vi "Separar ejes serial.vi"(8 "error in":errorcluster, 11 "Read buffer":string) -> (0 "error out":errorcluster, 1 "Pos Z":i32, 2 "Pos Y":i32, 3 "Pos X":i32)   [LabVIEW 2021]
panel:
  out "Eje Z":string
  out "Eje Y":string
  out "Eje X":string
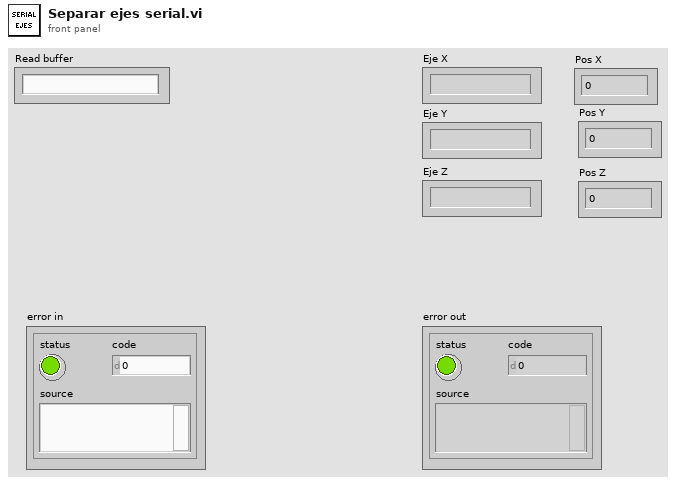
[diagram p1: front panel]
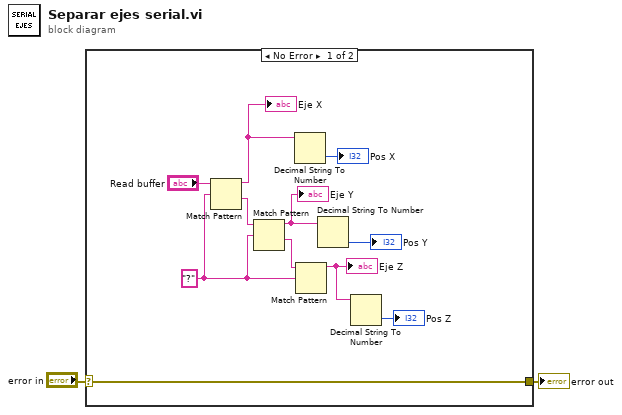
[diagram p0: block diagram]
diagram:
  n1 = case shown="No Error" "error in" {
    selector: "error in" -> [w13 w14]
    tunnel: [w13 w14] -> w1
    frame No Error {
      w9 = "?" ("regular expression")
      n2 = Match Pattern(string="Read buffer", regular expression=w9) -> (before substring=w8:string, after substring=w11:string)  [unwired: 1 in, 2 out]
      "Eje X" <- w8
      n3 = Match Pattern(string=w11, regular expression=w9) -> (before substring=w6:string, after substring=w10:string)  [unwired: 1 in, 2 out]
      "Eje Y" <- w6
      n4 = Decimal String To Number(string=w8) -> (number=→"Pos X":i32)  [unwired: 2 in, 1 out]
      n5 = Match Pattern(string=w10, regular expression=w9) -> (before substring=w5:string)  [unwired: 1 in, 3 out]
      "Eje Z" <- w5
      n6 = Decimal String To Number(string=w6) -> (number=→"Pos Y":i32)  [unwired: 2 in, 1 out]
      n7 = Decimal String To Number(string=w5) -> (number=→"Pos Z":i32)  [unwired: 2 in, 1 out]
    }
    frame Error {
    }
  }
  "error out" <- w1
